vi "Byte Value.vi"(1 "Length":i32, 2 "Offset":string, 3 "string":string) -> (0 "Value":i32)   [LabVIEW 2012]
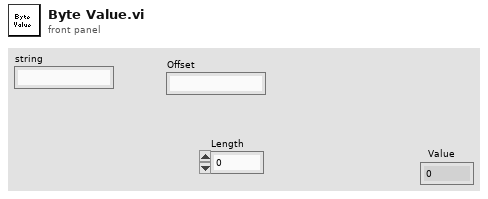
[diagram p1: front panel]
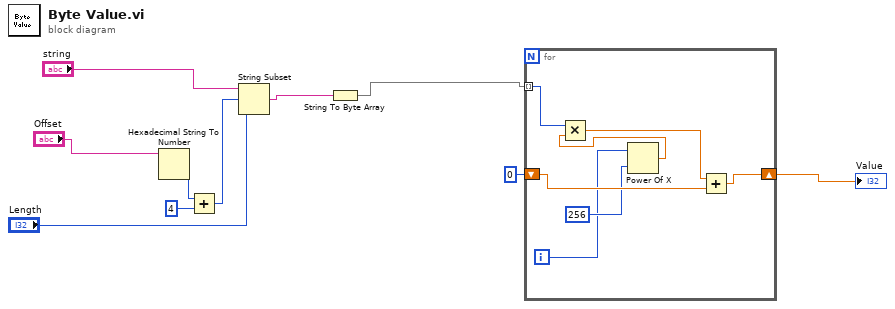
[diagram p0: block diagram]
diagram:
  n1 = Hexadecimal String To Number(string="Offset") -> (number=w8:u32)  [unwired: 2 in, 1 out]
  n2 = Add(x=w8, y=u32 4) -> (x+y=w6:u32)
  n3 = String Subset(string="string", offset (0)=w6, length (rest)="Length") -> (substring=w2:string)
  n4 = String To Byte Array(string=w2) -> (unsigned byte array=w5:u8[])
  n5 = for {
    tunnel: w5 -> [w17] mode=indexing
    shift-right: [w14] -> w3
    shift-left: 0 -> [w16]
    i -> [w11]
    n6 = Power Of X(1:256, 2:w11) -> (0:w13:dbl)
    n7 = Multiply(x=w17, y=w13) -> (x*y=w15:dbl)
    n8 = Add(x=w15, y=w16) -> (x+y=w14:dbl)
  }
  "Value" <- w3
